vi "Delete Stat Row.vi"(0 "StatBundle In":T1(array[cluster]), 11 "DeletedRow":string[](array[string])) -> (4 "StatBundle Out":T1(array[cluster]))   [LabVIEW 2013]
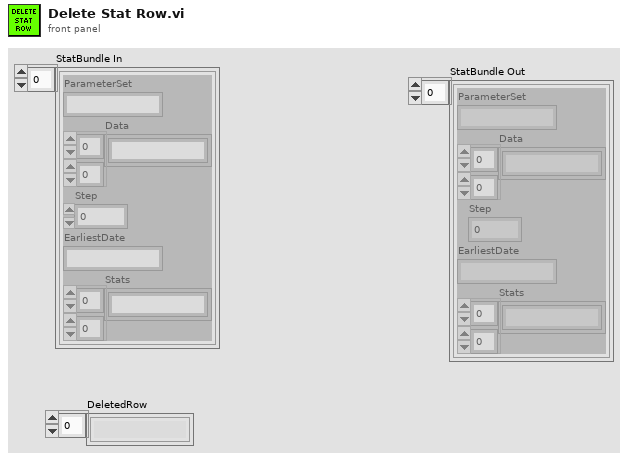
[diagram p1: front panel]
types:
  T1 = cluster{"ParameterSet":string, "Data":string[][], "Step":i32, "EarliestDate":string, "Stats":string[][]}[]
  T2 = typedef "Command Cluster.ctl" = cluster{"Para1":i32, "SP1":dbl, "Para2":i32, "SP2":dbl, "Para3":i32, "SP3":dbl}
  T3 = cluster{"ParameterSet":string, "Data":string[][], "Step":i32, "EarliestDate":string, "Stats":string[][]}
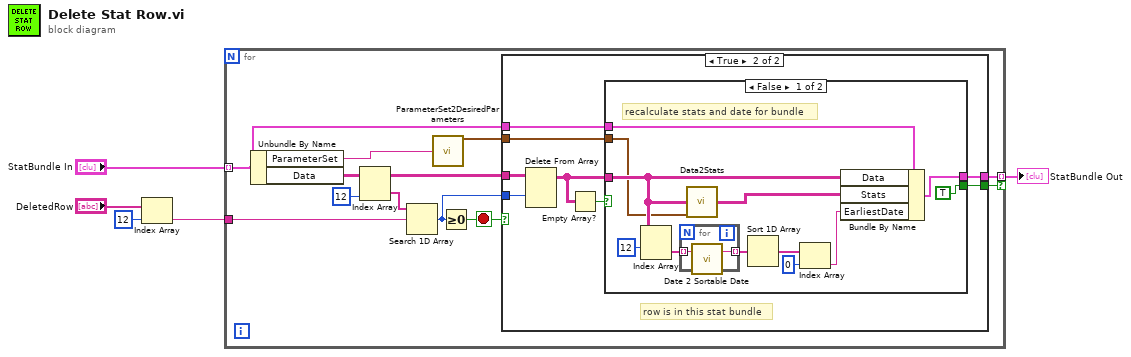
[diagram p0: block diagram]
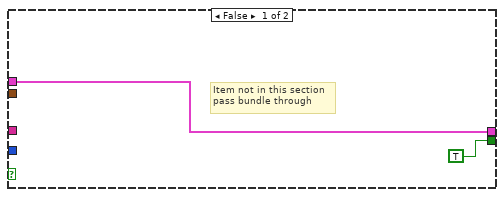
[diagram p2: hidden frame]
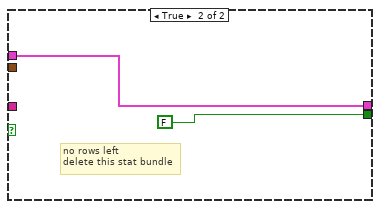
[diagram p3: hidden frame]
diagram:
  n1 = Index Array(array="DeletedRow", index=12) -> (element=w3:string)
  n2 = for {
    tunnel: "StatBundle In" -> [w8] mode=indexing
    tunnel: w3 -> [w14]
    tunnel: [w12] -> w1 mode=indexing if=w9
    stop <- w13 stop-if-true
    n3 = Unbundle By Name(w8) -> ("ParameterSet"=w7:string, "Data"=w10:string[][])
    n4 = Index Array(array=w10, index (col)=12 ("disabled index (col)")) -> (element=w15:string[])  [unwired: 1 in]
    n5 = Search 1D Array(1D array=w15, element=w14) -> (index of element=w11:i32)  [unwired: 1 in]
    n6 = call "ParameterSet2DesiredParameters.vi"("ParameterSet"=w7) -> ("DesiredParameters"=w6:T2)  [unwired: 14 in]
    n7 = Greater Or Equal To 0?(x=w11) -> (x >= 0?=w13:bool)
    n8 = case shown="True" w13 {
      tunnel: w8 -> [w18 w21]
      tunnel: [w18 w22] -> w12
      tunnel: w11 -> [_ w26]
      tunnel: w10 -> [_ w25]
      tunnel: [TRUE w23] -> w9
      tunnel: w6 -> [_ w19]
      frame False {
        # "Item not in this section\npass bundle through"
      }
      frame True {
        # "row is in this stat bundle"
        n9 = Delete From Array(array=w25, index (row)=w26) -> (array with subset deleted=w20:string[][])  [unwired: 2 in, 1 out]
        n10 = Empty Array?(array=w20) -> (empty?=w24:bool)
        n11 = case shown="False" w24 {
          tunnel: [TRUE FALSE] -> w23
          tunnel: [w29 w41] -> w22
          tunnel: w21 -> [w32 w41]
          tunnel: w20 -> [w31 _]
          tunnel: w19 -> [w27 _]
          frame False {
            # "recalculate stats and date for bundle"
            n12 = Index Array(array=w31, index (row)=12 ("index")) -> (element=w36:string[])  [unwired: 1 in]
            n13 = for {
              tunnel: w36 -> [w40] mode=indexing
              tunnel: [w39] -> w35 mode=indexing
              n14 = call "Date 2 Sortable Date.vi"("Date String"=w40) -> ("Sortable Date"=w39:string)  [unwired: 2 in]
            }
            n15 = call "Data2Stats.vi"("DataIn"=w31, "DesiredParameters"=w27) -> ("StatsOut"=w30:string[][])  [unwired: 13 in]
            n16 = Sort 1D Array(array=w35) -> (sorted array=w34:string[])
            n17 = Index Array(array=w34, index=0) -> (element=w28:string)
            n18 = Bundle By Name(cluster=w32, "Data"=w31, "Stats"=w30, "EarliestDate"=w28) -> (w29:T3)
          }
          frame True {
            # "no rows left\ndelete this stat bundle"
          }
        }
      }
    }
  }
  "StatBundle Out" <- w1
